vi "subGoVelEx.vi"(1 "AxisId":i32=1 min=1 max=6, 2 "Index":i32=1) -> ()   [LabVIEW 2020]
panel:
  in  "Start":bool
  in  "Speed":dbl caption="Speed [mm/s]" format="%.3f"
  in  "Close":bool
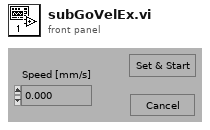
[diagram p1: front panel]
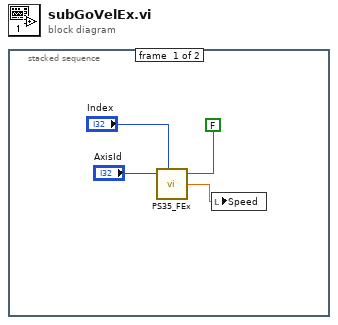
[diagram p0: block diagram]
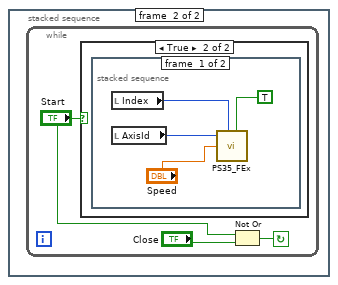
[diagram p2: hidden frame]
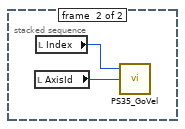
[diagram p4: hidden frame]
diagram:
  n1 = stacked-sequence {
    frame #0 {
      n2 = call "PS35_FEx.vi"("Axis number"="AxisId", "Control unit ID"="Index", "function"=FALSE ("WriteRead")) -> ("dValue-Out"=w4:dbl)  [unwired: 5 in, 1 out]
      n3 = local write "Speed"(w4) -> ()
    }
    frame #1 {
      n4 = while {
        stop <- w7 continue-if-true
        n5 = case shown="True" "Start" {
          frame False {
          }
          frame True {
            n6 = stacked-sequence {
              frame #0 {
                n7 = local read "Index"() -> (w8:i32)
                n8 = local read "AxisId"() -> (w10:i32)
                n9 = call "PS35_FEx.vi"("Axis number"=w10, "Control unit ID"=w8, "dValue-In"="Speed", "function"=TRUE ("WriteRead")) -> ()  [unwired: 4 in, 2 out]
              }
              frame #1 {
                n10 = local read "AxisId"() -> (w13:i32)
                n11 = local read "Index"() -> (w12:i32)
                n12 = call "PS35_GoVel.vi"("Axis number"=w13, "Control unit ID"=w12) -> ()  [unwired: 2 in, 1 out]
              }
            }
          }
        }
        n13 = Not Or(1:"Close", 2:"Start") -> (0:w7:bool)
      }
    }
  }
